vi "Tglobalvar.vi"() -> ()   [LabVIEW 2011]
panel:
  out "Tglobalvar":dbl
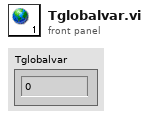
[diagram p1: front panel]
diagram:
